vi "ConnectToRobot.vi"(0 "error in":errorcluster, 1 "ip":string, 2 "SFTP Connect Parameters":refnum<k24>, 3 "Enable Dashboard":bool, 4 "Enable Primary Interface":bool, 5 "RTDE Connect Parameters":refnum<k24>) -> (14 "error out":errorcluster, 15 "UR Robot":refnum<k24>, 16 "Sftp":refnum<k24>, 17 "Dashboard":refnum<k24>, 18 "PrimaryInterface":refnum<k24>, 19 "Rtde":refnum<k24>)   [LabVIEW 2022 SP3, in "UnderAutomation.UniversalRobots.lvlib"]
uses:
  UnderAutomation.UniversalRobots.lvlib
  C:/Users/fg/Documents/UniversalRobots.vi/LabVIEW_2023/UnderAutomation.UniversalRobots/lib/UnderAutomation.UniversalRobots.dll
  LabVIEW_2023/UnderAutomation.UniversalRobots/lib/UnderAutomation.UniversalRobots.dll
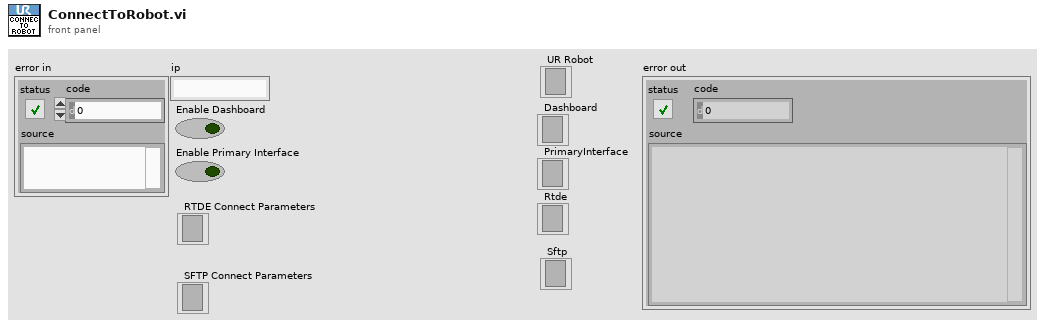
[diagram p1: front panel]
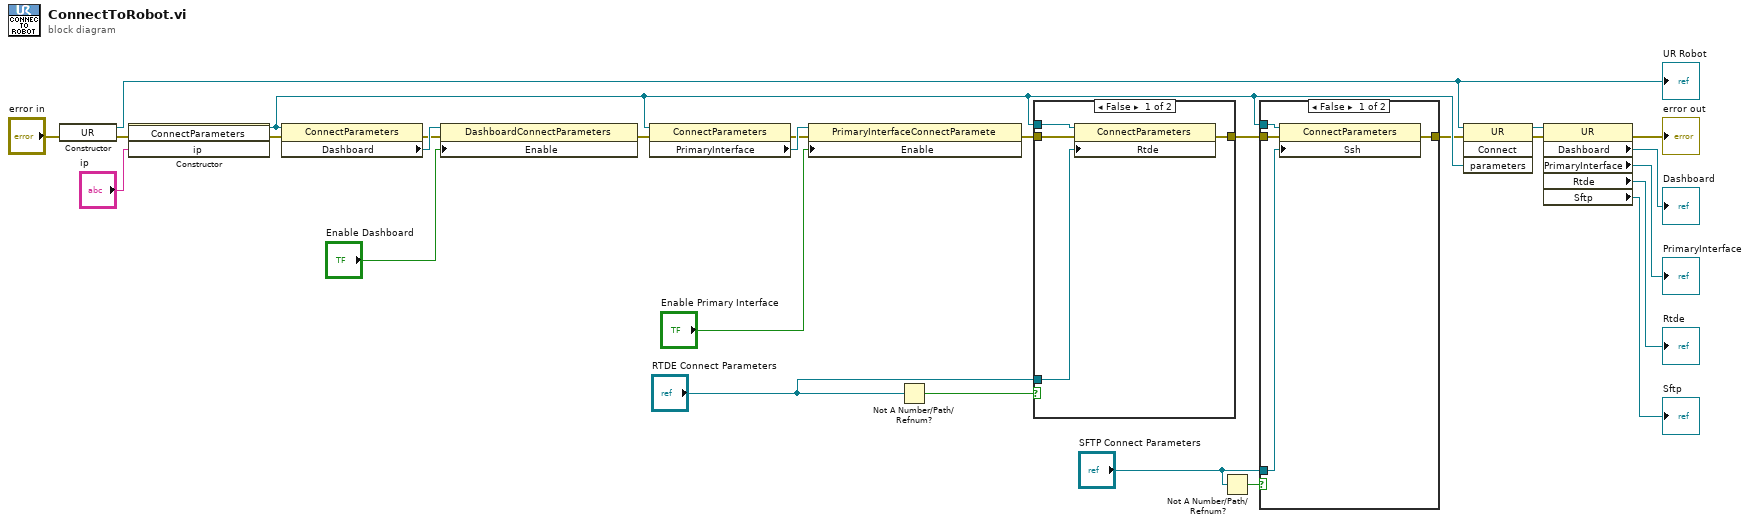
[diagram p0: block diagram]
diagram:
  n1 = constructor class="UR"(error in="error in") -> (reference out=w11:refnum<k24>, error out=w23:errorcluster)  [unwired: 2 in, 1 out]
  "UR Robot" <- w11
  n2 = constructor class="ConnectParameters"(error in=w23, "ip"="ip") -> (reference out=w9:refnum<k24>, error out=w22:errorcluster)  [unwired: 2 in, 2 out]
  n3 = property class="ConnectParameters"(reference=w9, error in=w22) -> (error out=w21:errorcluster, "Dashboard"=w25:refnum<k24>)  [unwired: 1 out]
  n4 = property class="DashboardConnectParameters"(reference=w25, error in=w21, "Enable"="Enable Dashboard") -> (error out=w20:errorcluster)  [unwired: 1 out]
  n5 = property class="ConnectParameters"(reference=w9, error in=w20) -> (error out=w19:errorcluster, "PrimaryInterface"=w24:refnum<k24>)  [unwired: 1 out]
  n6 = property class="PrimaryInterfaceConnectParamete"(reference=w24, error in=w19, "Enable"="Enable Primary Interface") -> (error out=w15:errorcluster)  [unwired: 1 out]
  n7 = Not A Number/Path/Refnum?(number/path/refnum="RTDE Connect Parameters") -> (NaN/Path/Refnum?=w17:bool)
  n8 = case shown="False" w17 {
    tunnel: w9 -> [w31 _]
    tunnel: "RTDE Connect Parameters" -> [w30 _]
    tunnel: w15 -> [w29 w32]
    tunnel: [w28 w32] -> w10
    frame False {
      n9 = property class="ConnectParameters"(reference=w31, error in=w29, "Rtde"=w30) -> (error out=w28:errorcluster)  [unwired: 1 out]
    }
    frame True {
    }
  }
  n10 = Not A Number/Path/Refnum?(number/path/refnum="SFTP Connect Parameters") -> (NaN/Path/Refnum?=w8:bool)
  n11 = case shown="False" w8 {
    tunnel: w9 -> [w36 _]
    tunnel: "SFTP Connect Parameters" -> [w35 _]
    tunnel: w10 -> [w34 w37]
    tunnel: [w33 w37] -> w6
    frame False {
      n12 = property class="ConnectParameters"(reference=w36, error in=w34, "Ssh"=w35) -> (error out=w33:errorcluster)  [unwired: 1 out]
    }
    frame True {
    }
  }
  n13 = invoke class="UR" method="Connect"(reference=w11, error in=w6, "parameters"=w9) -> (reference out=w12:refnum<k24>, error out=w2:errorcluster)  [unwired: 1 in, 2 out]
  n14 = property class="UR"(reference=w12, error in=w2) -> (error out=→"error out":errorcluster, "Dashboard"=→"Dashboard":refnum<k24>, "PrimaryInterface"=→"PrimaryInterface":refnum<k24>, "Rtde"=→"Rtde":refnum<k24>, "Sftp"=→"Sftp":refnum<k24>)  [unwired: 1 out]
